vi "quiz5.vi"() -> ()   [LabVIEW 2017]
panel:
  out "Mile":dbl format="%#.3g"
  out "kilometer":dbl format="%#_3g"
  out "meter":dbl format="%#_3g"
  out "Foot":dbl format="%#.3g"
  out "Finger":dbl format="%#.5g"
  out "min":dbl format="%#.6g"
  in  "Numeric":dbl
  # "mm"
  # "in"
  # "ft"
  # "m"
  # "Km"
  # "mi"
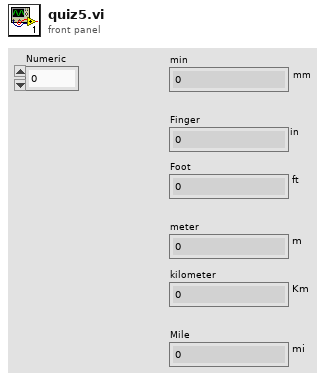
[diagram p1: front panel]
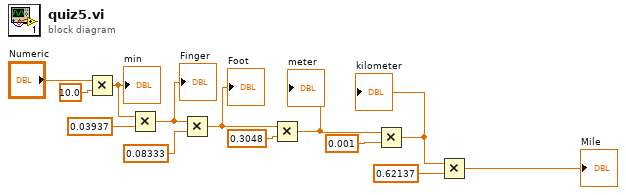
[diagram p0: block diagram]
diagram:
  n1 = Multiply(x="Numeric", y=10.0) -> (x*y=w10:dbl)
  "min" <- w10
  n2 = Multiply(x=w10, y=0.03937) -> (x*y=w8:dbl)
  "Finger" <- w8
  n3 = Multiply(x=w8, y=0.08333) -> (x*y=w6:dbl)
  "Foot" <- w6
  n4 = Multiply(x=w6, y=0.3048) -> (x*y=w4:dbl)
  "meter" <- w4
  n5 = Multiply(x=w4, y=0.001) -> (x*y=w2:dbl)
  "kilometer" <- w2
  n6 = Multiply(x=w2, y=0.62137) -> (x*y=→"Mile":dbl)
